vi "Center of Rect.vi"(3 "Grid Size":i32=5, 4 "Camera Center":cluster{"X":i32, "Y":i32}={"X"=160, "Y"=120}, 5 "Rectangle":T1) -> (1 "Grid Element":cluster{"X":i32, "Y":i32}={"X"=160, "Y"=120}, 2 "Center":cluster{dbl, dbl})   [LabVIEW 2011]
doc: "This VI computes the center of a Rectangle. Additionally,if a grid were overlayed on the camera lens, it computes which grid element (X,Y), this center would be in."
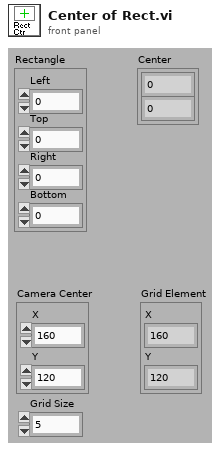
[diagram p1: front panel]
types:
  T1 = cluster{"Left":i32, "Top":i32, "Right":i32, "Bottom":i32}
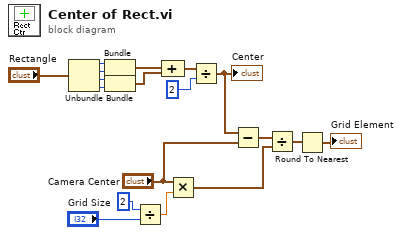
[diagram p0: block diagram]
diagram:
  n1 = Unbundle("Rectangle") -> ("Left"=w13:i32, "Top"=w14:i32, "Right"=w15:i32, "Bottom"=w16:i32)
  n2 = Bundle("Left"=w13, "Top"=w14) -> (w17:cluster{"Left":i32, "Top":i32})  [unwired: 1 out]
  n3 = Bundle("Right"=w15, "Bottom"=w16) -> (w18:cluster{"Right":i32, "Bottom":i32})  [unwired: 1 out]
  n4 = Divide(x=2, y="Grid Size") -> (x/y=w1:dbl)
  n5 = Compound Arithmetic op=ADD(w17, w18) -> (w11:cluster{i32, i32})
  n6 = Multiply(x="Camera Center", y=w1) -> (x*y=w6:cluster{"X":dbl, "Y":dbl})
  n7 = Divide(x=w11, y=2) -> (x/y=w9:cluster{dbl, dbl})
  "Center" <- w9
  n8 = Subtract(x=w9, y="Camera Center") -> (x-y=w7:cluster{dbl, dbl})
  n9 = Divide(x=w7, y=w6) -> (x/y=w5:cluster{dbl, dbl})
  n10 = Round To Nearest(number=w5) -> (nearest integer value=→"Grid Element":cluster{dbl, dbl})
